vi "QMH_Demo.vi"(11 "Sender":string="Demo") -> ()   [LabVIEW 2014]
panel:
  in  "Receiver":string="Demo_1"
  out "Receive data":string
  in  "Send data":string
  in  "STOP":bool
  in  "send":bool
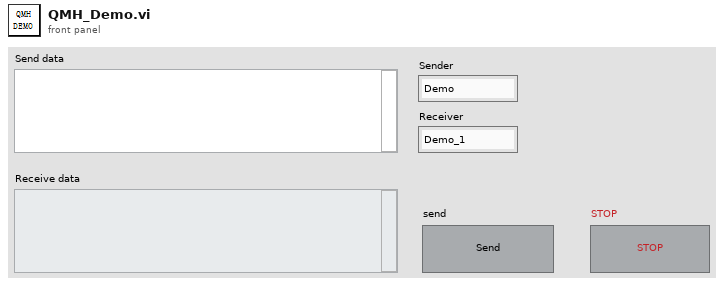
[diagram p1: front panel]
types:
  T1 = cluster{"Communication message":cluster{"Sender":string, "receiver":string, "message":string, "data":variant}, "Receive data":string}
  T2 = cluster{"Sender":string, "receiver":string, "message":string, "data":variant}
  T3 = enum32{"invalid app kind", "Development System", "Run Time System", "Student Edition", "Embedded LabVIEW", "Evaluation", "Custom"}
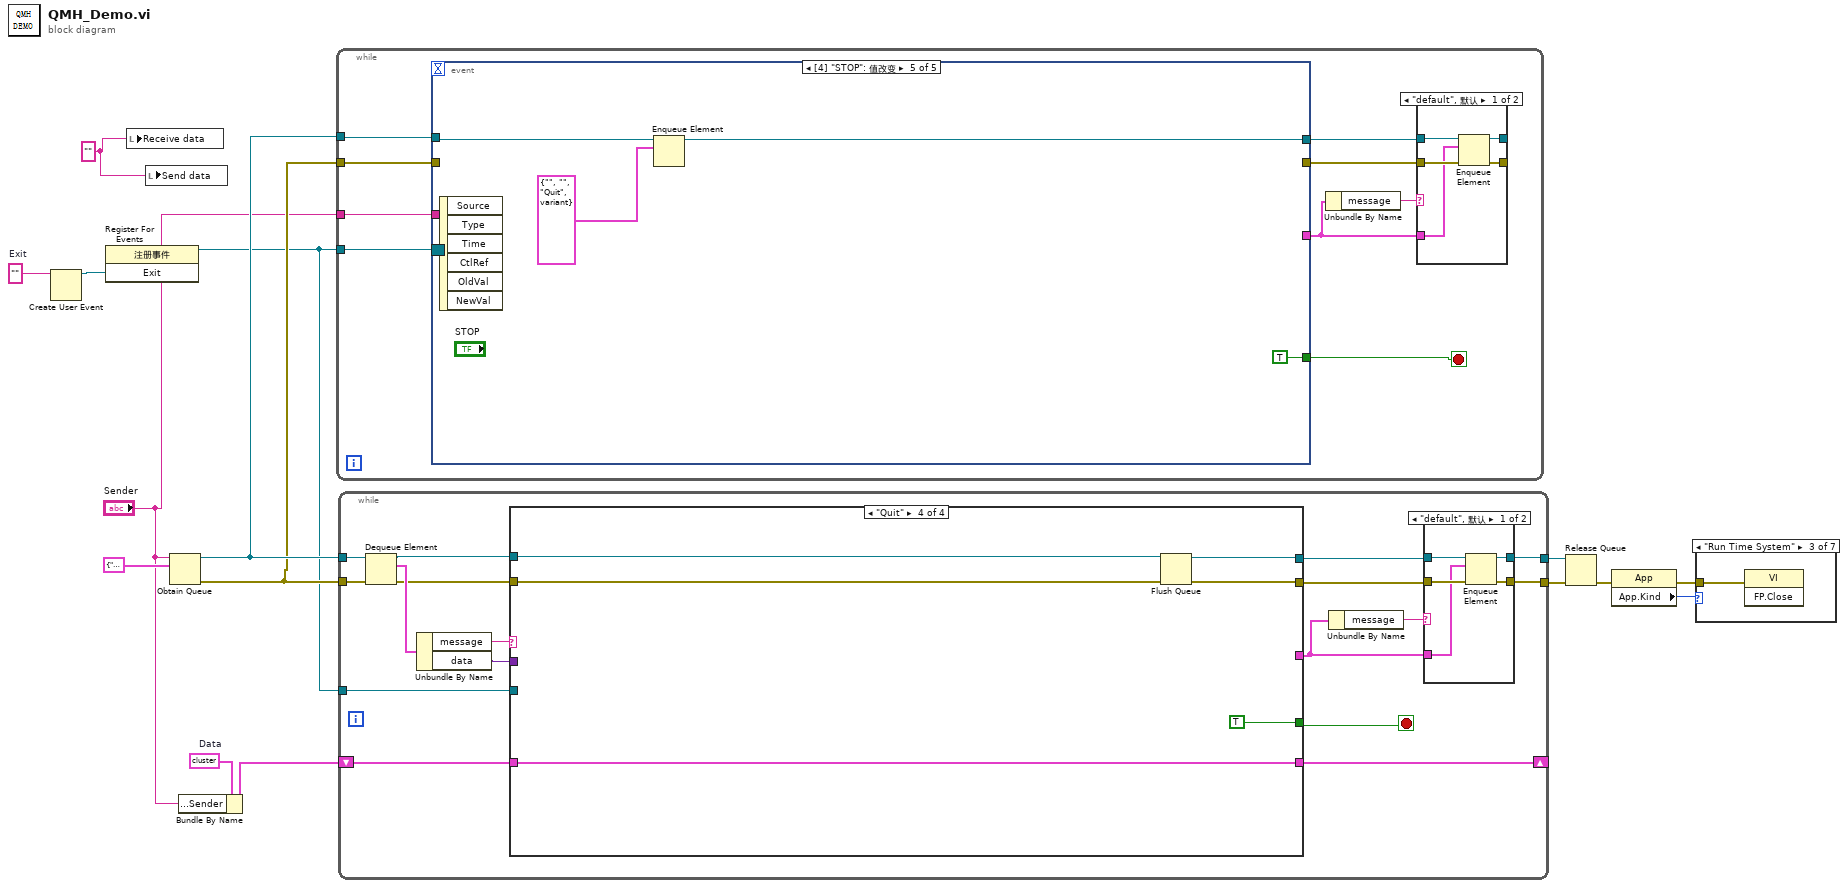
[diagram p0: block diagram]
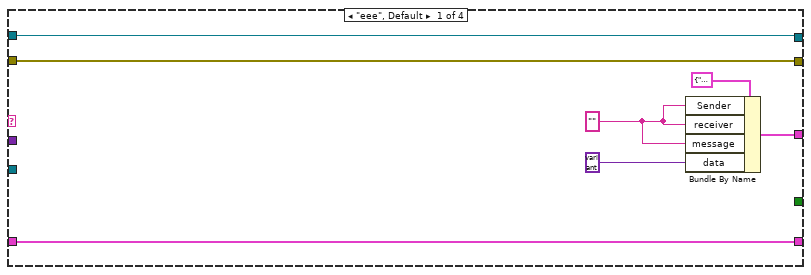
[diagram p9: hidden frame]
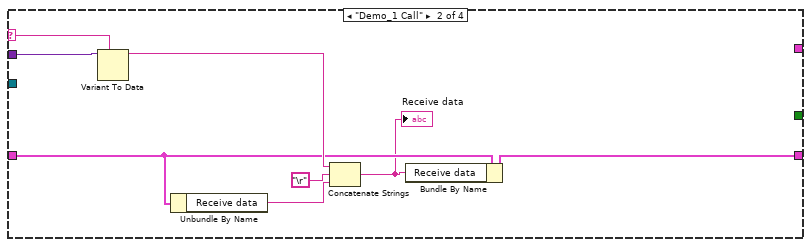
[diagram p10: hidden frame]
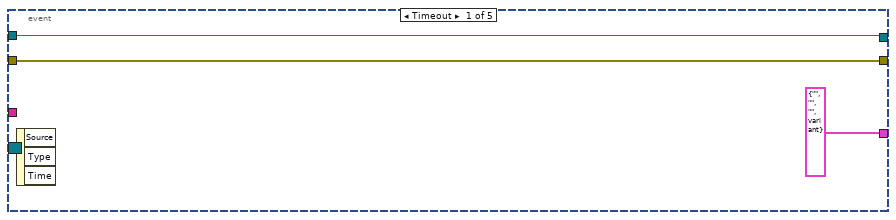
[diagram p13: hidden frame]
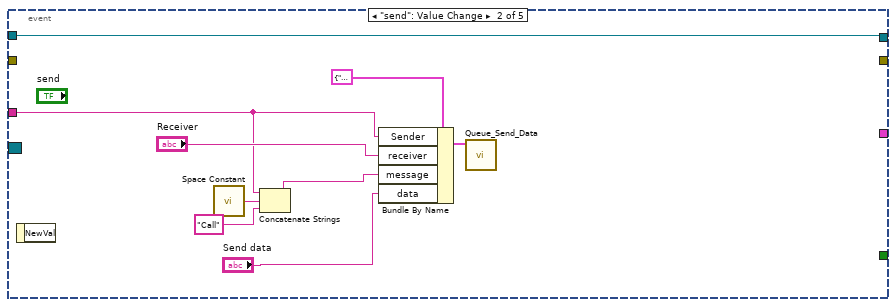
[diagram p14: hidden frame]
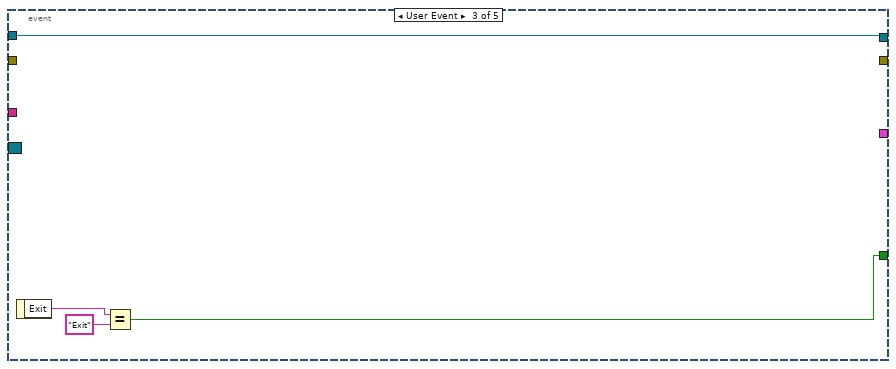
[diagram p15: hidden frame]
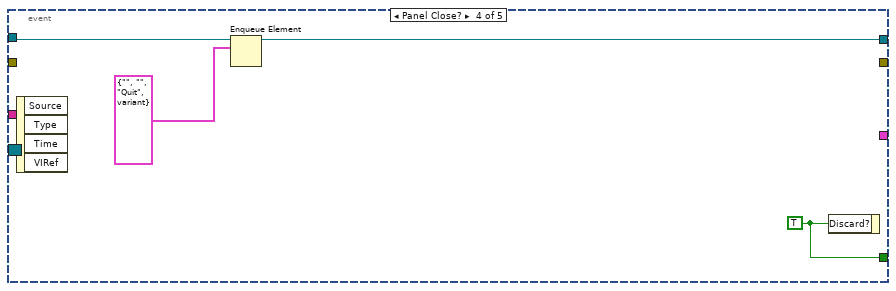
[diagram p16: hidden frame]
diagram:
  w2 = ""  # Exit
  w4 = ""
  w7 = T1 {"Communication message"={"Sender"="", "receiver"="", "message"="", "data"=variant}, "Receive data"=""}  # Data
  n1 = Create User Event(user event datatype=w2) -> (user event=w3:refnum<user-event>)  [unwired: 1 in, 1 out]
  n2 = register-events(w3) -> (reference out=w1:refnum<event-registration>)  [unwired: 2 in, 1 out]
  n3 = local write "Receive data"(w4) -> ()
  n4 = local write "Send data"(w4) -> ()
  n5 = Obtain Queue(name (unnamed)="Sender", element data type=T2 {"Sender"="", "receiver"="", "message"="", "data"=variant} ("Communication message")) -> (queue out=w15:refnum<queue>, error out=w8:errorcluster)  [unwired: 3 in, 1 out]
  n6 = Bundle By Name(cluster=w7, "Communication message.Sender"="Sender") -> (w6:T1)
  n7 = while {
    tunnel: w15 -> [w23]
    tunnel: w8 -> [w21]
    tunnel: "Sender" -> [w17]
    tunnel: w1 -> [w16]
    stop <- w24 stop-if-true
    n8 = event shown="[4] \"STOP\": 值改变" {
      selector: w16 -> [_ _ _ _ _]
      dyn-events: _ -> [_ _ _ _ _]
      timeout: _ -> [_ _ _ _ _]
      tunnel: [_ _ w44 w51 TRUE ("放弃？")] -> w24
      tunnel: w23 -> [w34 w43 w47 w50 w54]
      tunnel: [w34 w43 w47 w48 w52] -> w22
      tunnel: [T2 {"Sender"="", "receiver"="", "message"="", "data"=variant} ("Communication message") _ _ _ _] -> w19
      tunnel: [w33 _ _ _ _] -> w20
      tunnel: w21 -> [w33 _ _ _ _]
      tunnel: w17 -> [_ w37 _ _ _]
      event Timeout {
        n9 = event-data() -> ()  [unwired: 1 in, 3 out]
      }
      event "send": Value Change {
        n10 = event-data() -> ()  [unwired: 1 in, 1 out]
        n11 = call <vilib>:"Space Constant.vi"() -> ("String"=w36:string)
        n12 = Concatenate Strings(w37, w36, "Call" ("message")) -> (w38:string)
        n13 = Bundle By Name(cluster=T2 {"Sender"="", "receiver"="", "message"="", "data"=variant} ("Communication message"), "Sender"=w37, "receiver"="Receiver", "message"=w38, "data"="Send data") -> (w41:T2)
        n14 = call "Queue_Send_Data.vi"("Communication message"=w41) -> ()  [unwired: 10 in, 1 out]
      }
      event User Event {
        n15 = event-data() -> ("Exit"=w46:string)  [unwired: 1 in]
        n16 = Equal?(x=w46, y="Exit") -> (x = y?=w44:bool)
      }
      event Panel Close? {
        w51 = TRUE ("放弃？")
        n17 = event-data() -> ()  [unwired: 1 in, 4 out]
        n18 = Enqueue Element(queue=w50, element=T2 {"Sender"="", "receiver"="", "message"="Quit", "data"=variant} ("Communication message")) -> (queue out=w48:refnum<queue>)  [unwired: 2 in, 2 out]
        n19 = event-data("Discard?"=w51) -> ()  [unwired: 1 in, 1 out]
      }
      event "STOP": Value Change {
        n20 = event-data() -> ()  [unwired: 1 in, 6 out]
        n21 = Enqueue Element(queue=w54, element=T2 {"Sender"="", "receiver"="", "message"="Quit", "data"=variant} ("Communication message")) -> (queue out=w52:refnum<queue>)  [unwired: 2 in, 2 out]
      }
    }
    n22 = Unbundle By Name(w19) -> ("message"=w18:string)
    n23 = case shown="\"default\", 默认" w18 {
      tunnel: w22 -> [w29 w31]
      tunnel: w20 -> [w28 w30]
      tunnel: w19 -> [w27 _]
      tunnel: [w26 w31] -> _
      tunnel: [w25 w30] -> _
      frame "default", Default {
        n24 = Enqueue Element(queue=w29, element=w27, error in (no error)=w28) -> (queue out=w26:refnum<queue>, error out=w25:errorcluster)  [unwired: 1 in, 1 out]
      }
      frame "" {
      }
    }
  }
  n25 = while {
    tunnel: w15 -> [w72]
    tunnel: w8 -> [w71]
    tunnel: [w63] -> w14
    tunnel: [w62] -> w13
    shift-right: [w57] -> _
    shift-left: w6 -> [w58]
    tunnel: w1 -> [w56]
    stop <- w61 stop-if-true
    n26 = Dequeue Element(queue=w72, error in (no error)=w71) -> (queue out=w68:refnum<queue>, element=w70:T2, error out=w67:errorcluster)  [unwired: 1 in, 1 out]
    n27 = Unbundle By Name(w70) -> ("message"=w69:string, "data"=w64:variant)
    n28 = case shown="\"Quit\"" w69 {
      selector: w69 -> [_ w93 _ _]
      tunnel: [w86 _ w97 w102] -> w66
      tunnel: w68 -> [w86 _ w97 w101]
      tunnel: w67 -> [w85 _ w96 w99]
      tunnel: [w85 _ w96 w100] -> w65
      tunnel: w64 -> [_ w94 _ _]
      tunnel: [_ _ _ TRUE] -> w61
      tunnel: [w83 _ _ _] -> w60
      tunnel: [w80 w90 w95 w98] -> w57
      tunnel: w58 -> [w80 w89 w95 w98]
      tunnel: w56 -> [_ _ _ _]
      frame "eee", Default {
        w81 = ""
        n29 = Bundle By Name(cluster=T2 {"Sender"="", "receiver"="", "message"="", "data"=variant} ("Communication message"), "Sender"=w81, "receiver"=w81, "message"=w81, "data"=variant) -> (w83:T2)
      }
      frame "Demo_1 Call" {
        n30 = Variant To Data(type=w93, Variant=w94) -> (data=w92:string)  [unwired: 1 in, 1 out]
        n31 = Unbundle By Name(w89) -> ("Receive data"=w88:string)
        n32 = Concatenate Strings(w92, "\r", w88) -> (w87:string)
        "Receive data" <- w87
        n33 = Bundle By Name(cluster=w89, "Receive data"=w87) -> (w90:T1)
      }
      frame "Init" {
      }
      frame "Quit" {
        n34 = Flush Queue(queue=w101, error in (no error)=w99) -> (queue out=w102:refnum<queue>, error out=w100:errorcluster)  [unwired: 1 out]
      }
    }
    n35 = Unbundle By Name(w60) -> ("message"=w59:string)
    n36 = case shown="\"default\", 默认" w59 {
      tunnel: w66 -> [w77 w79]
      tunnel: w65 -> [w76 w78]
      tunnel: w60 -> [w75 _]
      tunnel: [w74 w79] -> w63
      tunnel: [w73 w78] -> w62
      frame "default", Default {
        n37 = Enqueue Element(queue=w77, element=w75, error in (no error)=w76) -> (queue out=w74:refnum<queue>, error out=w73:errorcluster)  [unwired: 1 in, 1 out]
      }
      frame "" {
      }
    }
  }
  n38 = Release Queue(queue=w14, error in (no error)=w13) -> (error out=w12:errorcluster)  [unwired: 1 in, 2 out]
  n39 = property class="App"(error in=w12) -> (error out=w11:errorcluster, "App.Kind"=w10:T3)  [unwired: 1 in, 1 out]
  n40 = case shown="\"Run Time System\"" w10 {
    tunnel: w11 -> [_ _ w104 _ _ _ _]
    frame "invalid app kind", Default {
    }
    frame "Development System" {
    }
    frame "Run Time System" {
      n41 = invoke class="VI" method="FP.Close"(error in=w104) -> ()  [unwired: 2 in, 3 out]
    }
    frame "Student Edition" {
    }
    frame "Embedded LabVIEW" {
    }
    frame "Evaluation" {
    }
    frame "Custom" {
    }
  }
